vi "2048_end.vi"(11 "Array in":i32[][](array[numeric])) -> (3 "Boolean":bool)   [LabVIEW 2022 SP3]
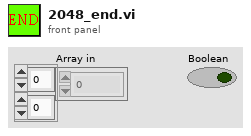
[diagram p1: front panel]
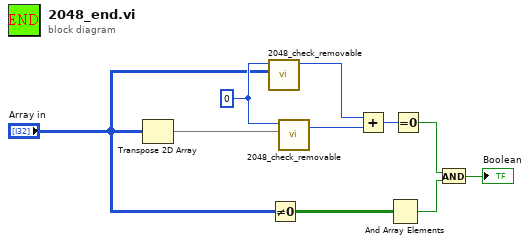
[diagram p0: block diagram]
diagram:
  w3 = 0
  n1 = Transpose 2D Array(2D array="Array in") -> (transposed array=w2:i32[][])
  n2 = call "2048_check_removable.vi"("Array in"="Array in", "Numeric in"=w3) -> ("Numeric out"=w5:i32)  [unwired: 8 in, 1 out]
  n3 = Not Equal To 0?(x="Array in") -> (x != 0?=w6:bool[][])
  n4 = call "2048_check_removable.vi"("Array in"=w2, "Numeric in"=w3) -> ("Numeric out"=w4:i32)  [unwired: 8 in, 1 out]
  n5 = Add(x=w5, y=w4) -> (x+y=w7:i32)
  n6 = And Array Elements(Boolean array=w6) -> (logical AND=w9:bool)
  n7 = Equal To 0?(x=w7) -> (x = 0?=w8:bool)
  n8 = And(x=w8, y=w9) -> (x .and. y?=→"Boolean":bool)
